vi "m10.wfg.05Click.vi"(1 "Param 0":dbl, 2 "Param 1":dbl, 3 "Param 2":dbl, 4 "Param 3":dbl, 5 "error in (no error)":errorcluster, 8 "Waveform Properties":T1={"Fs (Hz)"=20000.0, "Amplitude (V)"=5.0, "Ramp (s)"=0.02, "Duration (s)"=0.1} {"Ramp (s)" min=0.0; "Fs (Hz)" min=0.0}) -> (14 "Waveform Out":waveform(dbl), 19 "error out":errorcluster)   [LabVIEW 2013]
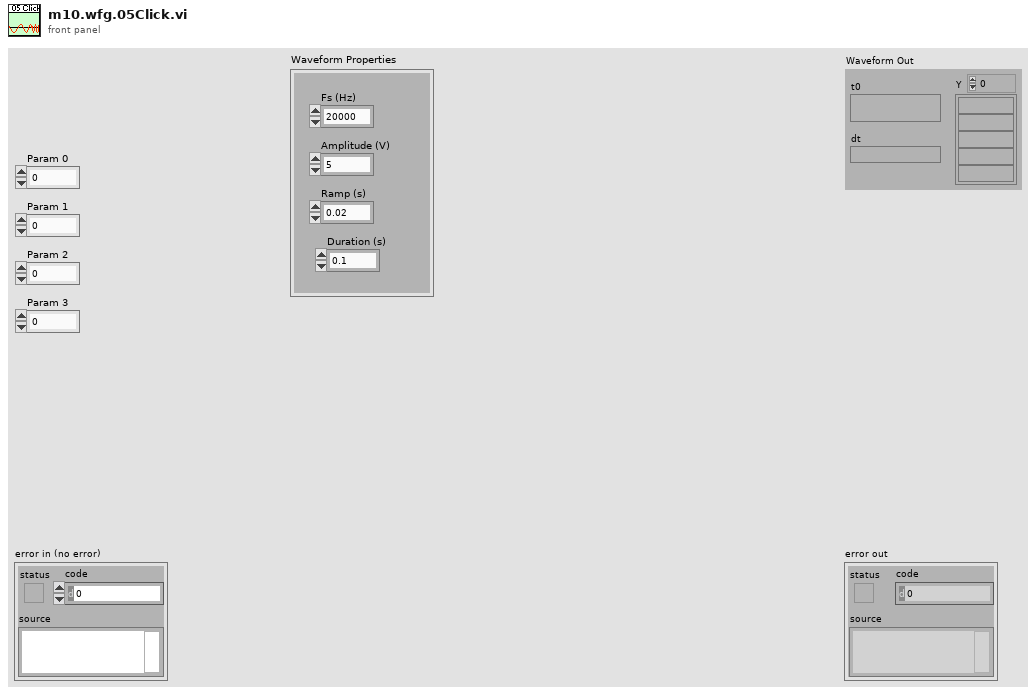
[diagram p1: front panel]
types:
  T1 = cluster{"Fs (Hz)":dbl, "Amplitude (V)":dbl, "Ramp (s)":dbl, "Duration (s)":dbl}
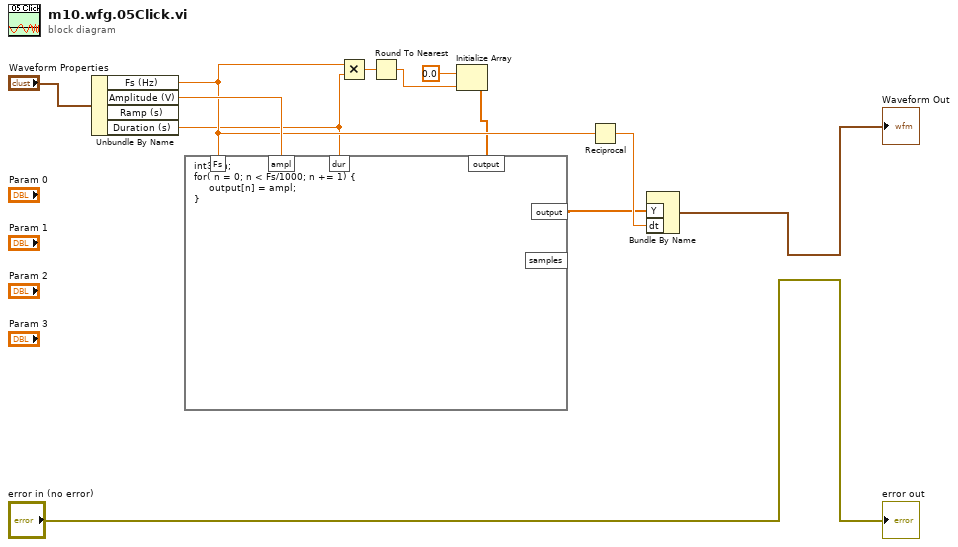
[diagram p0: block diagram]
diagram:
  n1 = Unbundle By Name("Waveform Properties") -> ("Fs (Hz)"=w7:dbl, "Amplitude (V)"=w11:dbl, "Duration (s)"=w3:dbl)  [unwired: 1 out]
  n2 = Multiply(x=w7, y=w3) -> (x*y=w6:dbl)
  n3 = Round To Nearest(number=w6) -> (nearest integer value=w5:dbl)
  n4 = Initialize Array(0.0 ("element"), w5) -> (w4:dbl[])
  n5 = formula code="int32 n;\nfor( n = 0; n < Fs/1000; n += 1) {\n     output[n] = ampl;\n}"("dur"=w3, "ampl"=w11, "Fs"=w7, "output"=w4) -> ("output"=w9:dbl[])  [unwired: 1 out]
  n6 = Reciprocal(x=w7) -> (1/x=w10:dbl)
  n7 = Bundle By Name("Y"=w9, "dt"=w10) -> (→"Waveform Out":waveform(dbl))  [unwired: 1 in]
  "error out" <- "error in (no error)"
